vi "Test Process Multiple Init.vi"(8 "error in (no error)":errorcluster, 11 "Process Test In":refnum<class "Process Dev Test.lvclass">) -> (0 "error out":errorcluster, 3 "Process Test Out":refnum<class "Process Dev Test.lvclass">)   [LabVIEW 2020, in "Process Dev Test.lvclass"]
uses:
  Process Dev Test.lvclass
  C:/Program Files (x86)/National Instruments/LabVIEW 2020/vi.lib/Astemes/LUnit/Test Case.lvclass
  <vilib>/Astemes/LUnit/Test Case.lvclass/Test Case.ctl
  <vilib>/Astemes/LUnit/LUnit Assertion Result.lvclass/LUnit Assertion Result.ctl
  <vilib>/Astemes/LUnit/LUnit Test Case Result.lvclass/LUnit Test Case Result.ctl
  <vilib>/Astemes/LUnit/LUnit Method Result.lvclass/LUnit Method Result.ctl
  source/Framework/Process/Process.lvclass/Process.ctl
  <vilib>/Astemes/LUnit/Palette/Fail.vi
  <vilib>/Astemes/LUnit/Palette/Pass.vi
  <vilib>/Astemes/LUnit/Set Assertion Type.vi
  source/Framework/Process/Private/SubVIs/Wait for finish.vi
  source/Framework/Process/Protected/Messaging/Enqueue Message.vi
  source/Framework/Process/Private/SubVIs/Set Lifecycle State.vi
  source/Framework/Process/Public/Lifecycle/Get Lifecycle State.vi
  <vilib>/Astemes/LUnit/Add test result.vi
  <vilib>/Astemes/LUnit/LUnit Write Passed.vi
  <vilib>/Astemes/LUnit/LUnit Write Message.vi
  <vilib>/Astemes/LUnit/LUnit Write Description.vi
  <vilib>/Astemes/LUnit/LUnit Write Assertion Type.vi
  source/Framework/Process/Private/SubVIs/Handle Debug Data.vi
  <vilib>/Utility/error.llb/Clear Errors.vi
  <vilib>/Astemes/LUnit/LUnit Record Assertion Result.vi
  source/Framework/Logging/Log Debug.vi
  <vilib>/AdvancedString/1D String Array to Delimited String.vi
  <vilib>/Utility/High Resolution Relative Seconds.vi
  <vilib>/Astemes/LUnit/LUnit Aggregate Assertion Results.vi
  <vilib>/Astemes/LUnit/Assertion Result/LUnit Read Status.vi
  <vilib>/Astemes/LUnit/LUnit Read Message.vi
  <vilib>/Astemes/LUnit/LUnit Read Description.vi
  <vilib>/Astemes/LUnit/Method Result/LUnit Merge Status.vi
  <vilib>/Astemes/LUnit/LUnit Concatenate result strings.vi
  <vilib>/Utility/error.llb/Error Cluster From Error Code.vi
  source/Framework/Process/Public/Read Name.vi
  <vilib>/Astemes/LUnit/LUnit Assertion Result.lvclass
  source/Framework/Process/Process.lvclass
  <vilib>/Astemes/LUnit/Test Case.lvclass
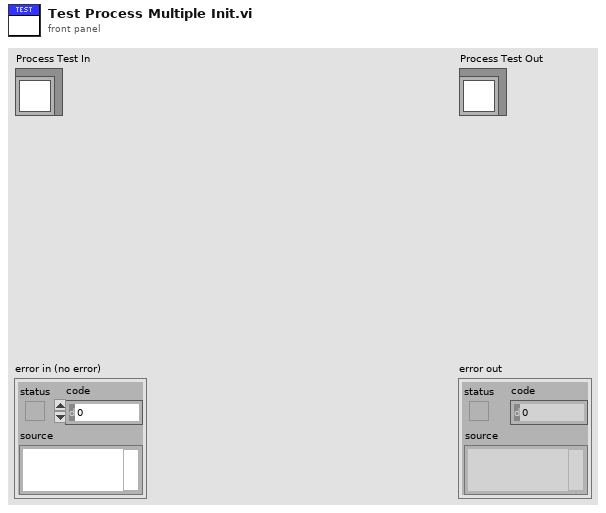
[diagram p1: front panel]
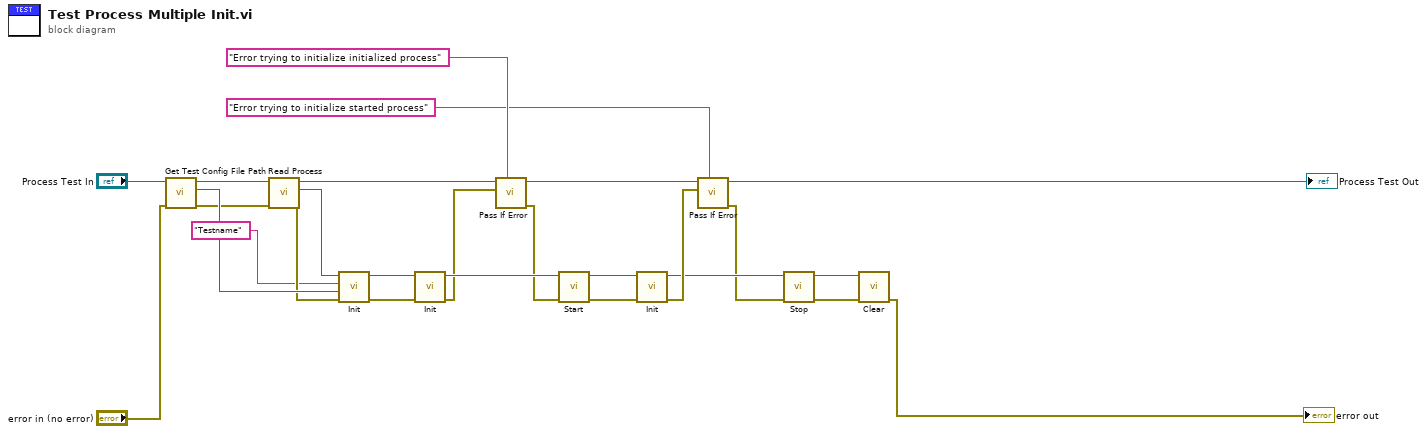
[diagram p0: block diagram]
diagram:
  n1 = call "Get Test Config File Path.vi"("error in (no error)"="error in (no error)", "Process Test In"="Process Test In") -> ("error out"=w18:errorcluster, "Test config path"=w21:path, "Process Test Out"=w23:refnum<class "Process Dev Test.lvclass">)  [unwired: 7 in]
  n2 = call "Read Process.vi"("error in (no error)"=w18, "Process Test in"=w23) -> ("error out"=w19:errorcluster, "Process.lvclass"=w20:refnum<class "Process.lvclass">, "Process Test out"=w13:refnum<class "Process Dev Test.lvclass">)  [unwired: 7 in]
  n3 = call-dynamic "Init.vi"("error in (no error)"=w19, "Config File Path"=w21, "Name"="Testname", "Process In"=w20) -> ("error out"=w15:errorcluster, "Process Out"=w24:refnum<class "Process.lvclass">)  [unwired: 6 in]
  n4 = call-dynamic "Init.vi"("error in (no error)"=w15, "Process In"=w24) -> ("error out"=w11:errorcluster, "Process Out"=w26:refnum<class "Process.lvclass">)  [unwired: 8 in]
  n5 = call <vilib>:"Pass If Error.vi"("Description"="Error trying to initialize initialized process", "Assert error"=w11, "LUnit Test Case In"=w13) -> ("error out"=w10:errorcluster, "LUnit Test Case Out"=w5:refnum<class "Process Dev Test.lvclass">)  [unwired: 7 in]
  n6 = call "Start.vi"("error in (no error)"=w10, "Process In"=w26) -> ("error out"=w12:errorcluster, "Process Out"=w7:refnum<class "Process.lvclass">)  [unwired: 7 in, 1 out]
  n7 = call-dynamic "Init.vi"("error in (no error)"=w12, "Process In"=w7) -> ("error out"=w8:errorcluster, "Process Out"=w6:refnum<class "Process.lvclass">)  [unwired: 8 in]
  n8 = call <vilib>:"Pass If Error.vi"("Description"="Error trying to initialize started process", "Assert error"=w8, "LUnit Test Case In"=w5) -> ("error out"=w2:errorcluster, "LUnit Test Case Out"=→"Process Test Out":refnum<class "Process Dev Test.lvclass">)  [unwired: 7 in]
  n9 = call "Stop.vi"("error in (no error)"=w2, "Process In"=w6) -> ("error out"=w16:errorcluster, "Process Out"=w17:refnum<class "Process.lvclass">)  [unwired: 7 in, 1 out]
  n10 = call-dynamic "Clear.vi"("error in (no error)"=w16, "Process In"=w17) -> ("error out"=→"error out":errorcluster)  [unwired: 9 in]
